vi "Interrogate_register.vi"(6 "Address override":i32, 8 "error in (no error)":errorcluster, 9 "UUT Index":i32, 10 "Register mutli-protocol location":T2={"General Parameter name"="", "MODBUS Register"=0, "Profibus"={"Friendly name"="", "PA"={"Slot"=0, "Index"=0}, "DP"={"Slot"=0, "Index"=0}, "Tag"=""}, "Fieldbus"={"Parameter name"="", "Fieldbus Block"="", "Fieldbus Tag"=""}, "data type"=enum."float", "DeviceNET"={"ClassId"=102, "InstanceId"=1, "AttributeId"=12}, "Cluster"={"address"=0, "Mode"=0}, "Length"=0} {"Cluster"."Mode" items=["None", "MODBUS", "HART", "Profibus DP", "Profibus PA", "Fieldbus", "DeviceNET"]}, 11 "PROFIBUS in":refnum<class "Profibus.lvclass">) -> (0 "error out":errorcluster, 1 "Parameter name":string, 2 "output":sgl, 3 "PROFIBUS out":refnum<class "Profibus.lvclass">, 4 "output cluster":T1)   [LabVIEW 2016, in "Profibus.lvclass"]
uses:
  Profibus.lvclass
  Typedef/comm_variable_definition.ctl
  Typedef/Comm_mode_and_address_type.ctl
  Typedef/Comm_mode_type_combo.ctl
  Profibus VISA Driver/DF PROFI II.llb/CS_PB_DPV1_MSAC2_ReadReqData.ctl
  Profibus.lvclass/Profibus.ctl
  Protocol Class/Protocol.lvclass
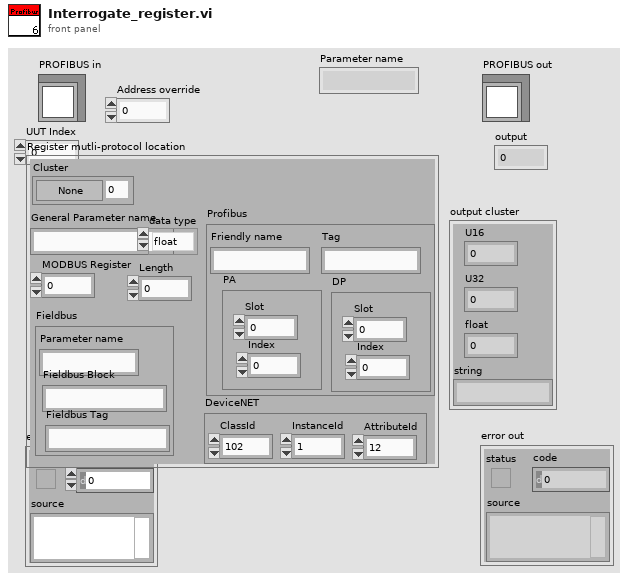
[diagram p1: front panel]
types:
  T1 = cluster{"U16":u16, "U32":u32, "float":sgl, "string":string}
  T2 = typedef "comm_variable_definition.ctl" = cluster{"General Parameter name":string, "MODBUS Register":i32, "Profibus":cluster{"Friendly name":string, "PA":cluster{"Slot":i32, "Index":i32}, "DP":cluster{"Slot":i32, "Index":i32}, "Tag":string}, "Fieldbus":cluster{"Parameter name":string, "Fieldbus Block":string, "Fieldbus Tag":string}, "data type":enum16{"float", "UINT", "UINT32", "STRING"}, "DeviceNET":cluster{"ClassId":u16, "InstanceId":u16, "AttributeId":u8}, "Cluster":T3, "Length":i32}
  T3 = typedef "Comm_mode_and_address_type.ctl" = cluster{"address":i32, "Mode":T4}
  T4 = typedef "Comm_mode_type_combo.ctl" = u16
  T5 = typedef "CS_PB_DPV1_MSAC2_ReadReqData.ctl" = cluster{"Communication ref.:":u8, "Slot number:":u8, "Index:":u8, "Length:":u8}
  T6 = enum16{"Boolean", "Int8", "Unsigned8", "Int16", "Unsigned16", "Int32", "Unsigned32", "Float"}
  T7 = cluster{"Device address":i32, "Switch index":i32, "Communication ref.:":u8}[]
  T8 = cluster{"Friendly name":string, "PA":cluster{"Slot":i32, "Index":i32}, "DP":cluster{"Slot":i32, "Index":i32}, "Tag":string}
  T9 = cluster{"Device address":i32, "Switch index":i32, "Communication ref.:":u8}
  T10 = typedef "CS_PB_DPV1_MSAC2_ReadConData.ctl" = cluster{"Communication ref.:":u8, "Length:":u8, "Data:":u8[]}
  T11 = typedef "CS_PB_DPV1_AbortIndData.ctl" = cluster{"Remote address:":u8, "Response SAP:":u8, "Locally generated":bool, "Subnet:":u8, "Instance:":u8, "Reasoncode:":u8, "Additional detail:":u16}
  T12 = typedef "CS_PB_DPV1_ErrorData.ctl" = cluster{"Communication ref.:":u8, "Remote address:":u8, "Error decode:":u8, "Error code 1:":u8, "Error code 2:":u8}
  T13 = cluster{"Read data":T10, "Abort data":T11, "Error data":T12}
  T14 = cluster{"Error":bool, "Status":i32, "Info":string}
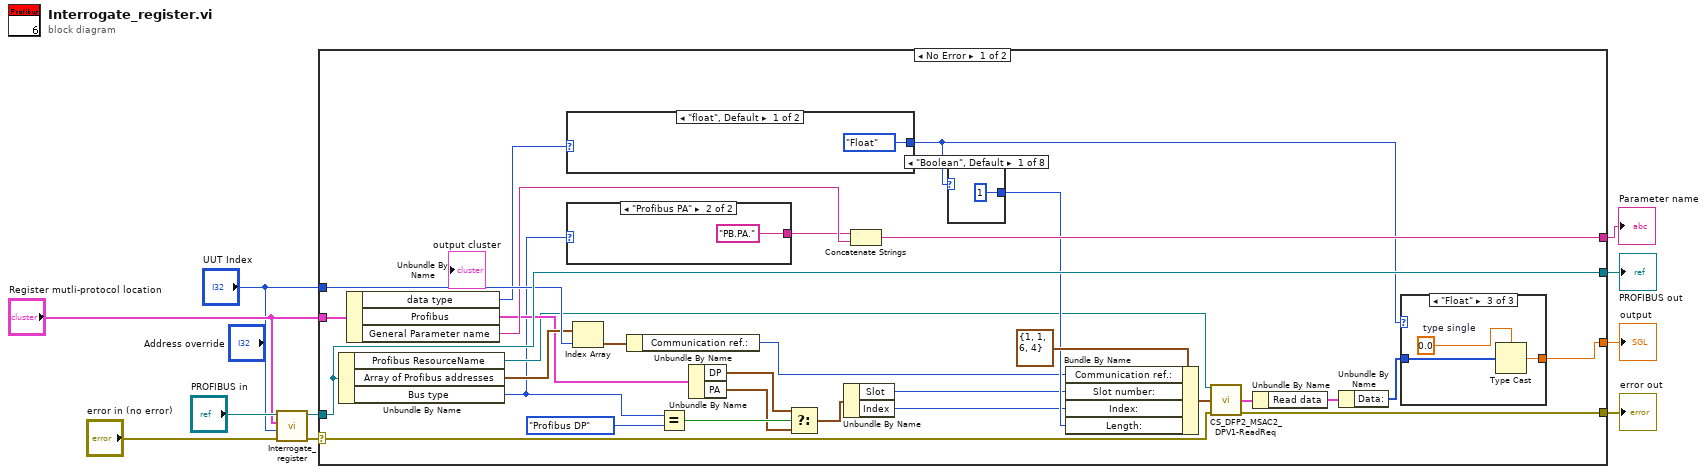
[diagram p0: block diagram]
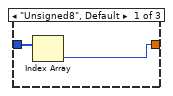
[diagram p2: hidden frame]
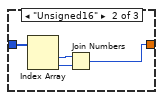
[diagram p3: hidden frame]
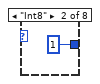
[diagram p4: hidden frame]
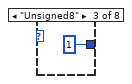
[diagram p5: hidden frame]
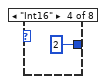
[diagram p6: hidden frame]
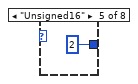
[diagram p7: hidden frame]
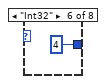
[diagram p8: hidden frame]
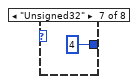
[diagram p9: hidden frame]
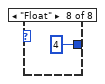
[diagram p10: hidden frame]
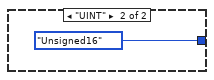
[diagram p11: hidden frame]
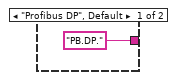
[diagram p12: hidden frame]
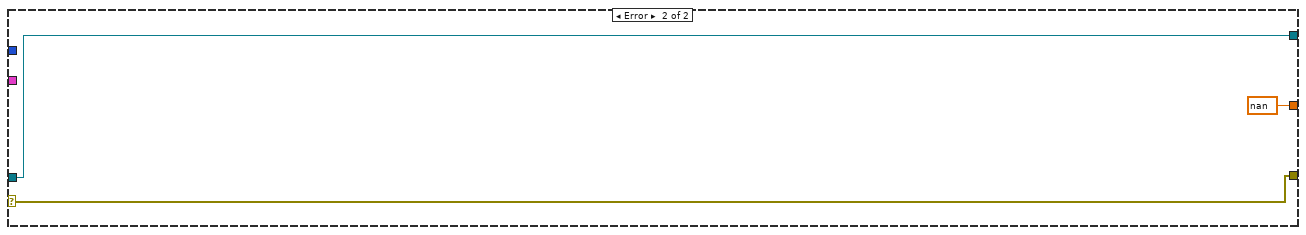
[diagram p13: hidden frame]
diagram:
  n1 = call-parent "Interrogate_register.vi"("error in (no error)"="error in (no error)", "UUT Index"="UUT Index", "Register mutli-protocol location"="Register mutli-protocol location", "Protocol in"="PROFIBUS in") -> ("error out"=w8:errorcluster, "Protocol out"=w7:refnum<class "Profibus.lvclass">)  [unwired: 3 in, 3 out]
  n2 = case shown="No Error" w8 {
    selector: w8 -> [w11 w64]
    tunnel: "Register mutli-protocol location" -> [w40 _]
    tunnel: [w13 sgl nan ("type single")] -> w2
    tunnel: [w12 w64] -> w3
    tunnel: "UUT Index" -> [w38 _]
    tunnel: w7 -> [w39 w62]
    tunnel: [w39 w62] -> w4
    tunnel: [w35 _] -> w1
    frame No Error {
      n3 = Unbundle By Name(w39) -> ("Profibus ResourceName"=w24:refnum<visa-resource-name>, "Array of Profibus addresses"=w34:T7, "Bus type"=w21:enum16{"Profibus DP", "Profibus PA"})
      n4 = Unbundle By Name(w40) -> ("data type"=w33:enum16{"float", "UINT", "UINT32", "STRING"}, "Profibus"=w27:T8, "General Parameter name"=w37:string)
      n5 = case shown="\"float\", Default" w33 {
        tunnel: [T6."Float" ("Type") T6."Unsigned16" ("Type")] -> w30
        frame "float", Default {
        }
        frame "UINT" {
        }
      }
      n6 = case shown="\"Profibus PA\"" w21 {
        tunnel: ["PB.DP." ("Protocol name") "PB.PA." ("Protocol name")] -> w36
        frame "Profibus DP", Default {
        }
        frame "Profibus PA" {
        }
      }
      n7 = Index Array(array=w34, index=w38) -> (element=w15:T9)
      n8 = Unbundle By Name(w15) -> ("Communication ref.:"=w14:u8)
      n9 = Equal?(x=w21, y=enum16{"Profibus DP", "Profibus PA"}."Profibus DP" ("Bus type")) -> (x = y?=w23:bool)
      n10 = Unbundle By Name(w27) -> ("DP"=w20:cluster{"Slot":i32, "Index":i32}, "PA"=w19:cluster{"Slot":i32, "Index":i32})
      n11 = Select(t=w20, s=w23, f=w19) -> (s? t:f=w18:cluster{"Slot":i32, "Index":i32})
      n12 = Unbundle By Name(w18) -> ("Slot"=w17:i32, "Index"=w16:i32)
      n13 = Concatenate Strings(w36, w37) -> (w35:string)
      n14 = case shown="\"Boolean\", Default" w30 {
        tunnel: [u8 1 ("Length:") u8 1 ("Length:") u8 1 ("Length:") u8 2 ("Length:") u8 2 ("Length:") u8 4 ("Length:") u8 4 ("Length:") u8 4 ("Length:")] -> w26
        frame "Boolean", Default {
        }
        frame "Int8" {
        }
        frame "Unsigned8" {
        }
        frame "Int16" {
        }
        frame "Unsigned16" {
        }
        frame "Int32" {
        }
        frame "Unsigned32" {
        }
        frame "Float" {
        }
      }
      n15 = Bundle By Name(cluster=T5 {"Communication ref.:"=1, "Slot number:"=1, "Index:"=6, "Length:"=4} ("Read data"), "Communication ref.:"=w14, "Slot number:"=w17, "Index:"=w16, "Length:"=w26) -> (w25:T5)
      n16 = call "CS_DFP2_MSAC2_DPV1-ReadReq.vi"("DFP2 resource name"=w24, "Read data"=w25, "Error in:"=w11) -> ("DPV1-Read"=w31:T13, "Error out:"=w12:T14)  [unwired: 9 in, 2 out]
      n17 = Unbundle By Name(w31) -> ("Read data"=w32:T10)
      n18 = Unbundle By Name(w32) -> ("Data:"=w29:u8[])
      n19 = case shown="\"Float\"" w30 {
        tunnel: w29 -> [w42 w46 w48]
        tunnel: [w41 w43 w47] -> w13
        frame "Unsigned8", Default {
          n20 = Index Array(array=w42) -> (element=w41:u8)  [unwired: 1 in]
        }
        frame "Unsigned16" {
          n21 = Index Array(array=w46) -> (element #1=w45:u8, element #2=w44:u8)  [unwired: 2 in]
          n22 = Join Numbers(hi=w45, lo=w44) -> ((hi.lo)=w43:u16)
        }
        frame "Float" {
          w49 = sgl 0.0  # type single
          n23 = Type Cast(type=w49, x=w48) -> (*(type *) &x=w47:sgl)
        }
      }
    }
    frame Error {
    }
  }
  "error out" <- w3
  "PROFIBUS out" <- w4
  "output" <- w2
  "Parameter name" <- w1
